vi "Read SlideData.vi"(8 "error in (no error)":errorcluster, 11 "Game in":refnum<class "Game.lvclass">) -> (0 "error out":errorcluster, 2 "SlideData":T1={"updown_buffer"=[], "Speed"=10.0, "CurrPos"={"x"=0.0, "y"=0.0}, "TargetPos"={"x"=0.0, "y"=0.0}, "TempDistance"={"x"=0.0, "y"=0.0}, "leftright_buffer"=[], "doPush_leftright"=FALSE}, 3 "Game out":refnum<class "Game.lvclass">)   [LabVIEW 2019, in "RT_Game.lvlib" / "Game.lvclass"]
uses:
  Game.lvclass
  SlideData.ctl
  ScreenSide.ctl
  Coordinate.ctl
  SlideJob.ctl
  Game.lvclass/Game.ctl
  Engine/Engine.lvclass
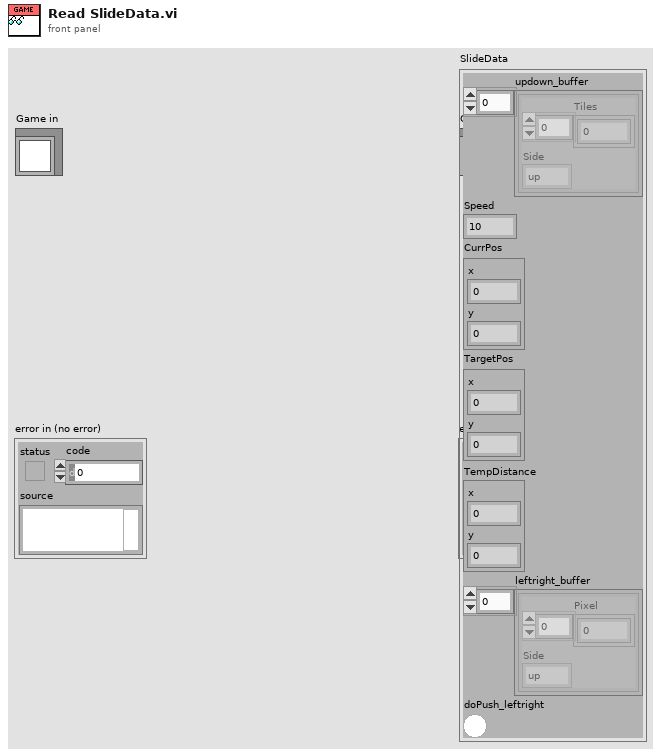
[diagram p1: front panel]
types:
  T1 = typedef "RT_Game.lvlib/Game.lvclass/SlideData.ctl" = cluster{"updown_buffer":cluster{"Tiles":u32[], "Side":T2}[], "Speed":dbl, "CurrPos":T3, "TargetPos":T3, "TempDistance":T3, "leftright_buffer":T4[], "doPush_leftright":bool}
  T2 = typedef "RT_Game.lvlib/Game.lvclass/ScreenSide.ctl" = enum16{"up", "down", "left", "right"}
  T3 = typedef "RT_Game.lvlib/Game.lvclass/Coordinate.ctl" = cluster{"x":dbl, "y":dbl}
  T4 = typedef "RT_Game.lvlib/Engine.lvclass/SlideJob.ctl" = cluster{"Pixel":u32[], "Side":T2}
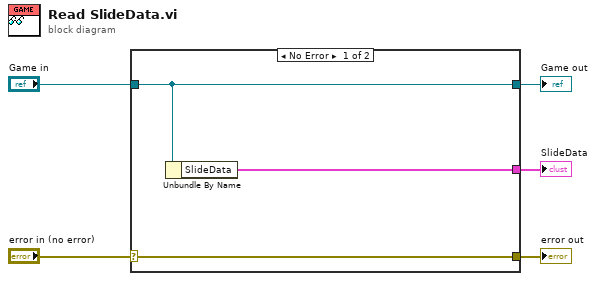
[diagram p0: block diagram]
diagram:
  n1 = case shown="No Error" "error in (no error)" {
    selector: "error in (no error)" -> [w8 w9]
    tunnel: [w8 w9] -> w4
    tunnel: [w7 w10] -> w2
    tunnel: "Game in" -> [w7 w10]
    tunnel: [w6 _] -> w1
    frame No Error {
      n2 = Unbundle By Name(w7) -> ("SlideData"=w6:T1)
    }
    frame Error {
    }
  }
  "error out" <- w4
  "Game out" <- w2
  "SlideData" <- w1
